vi "SequenceStatus.vi"(8 "error in (no error)":errorcluster, 9 "Motion Stopped":bool, 11 "VXMMotionManager in":refnum<class "VXMMotionManager.lvclass">) -> (0 "error out":errorcluster, 1 "last axis = True":bool, 3 "VXMMotionManager out":refnum<class "VXMMotionManager.lvclass">)   [LabVIEW 2019, in "VXMMotionManager.lvclass"]
doc: "change state from monitor motion to start next move\nincrement axis"
uses:
  VXMMotionManager.lvclass
  MoveAllAbsoluteStates.ctl
  VXMMotionManager.lvclass/VXMMotionManager.ctl
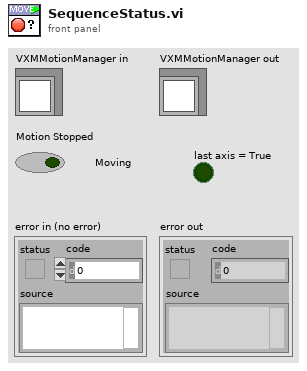
[diagram p1: front panel]
types:
  T1 = typedef "VXMMotionManager.lvclass/MoveAllAbsoluteStates.ctl" = enum16{"start next move", "wait motion end"}
  T2 = typedef "singleAxisMoveDef.ctl" = cluster{"mmWave Axis":T3, "eng. value":dbl}
  T3 = typedef "mmWaveAxis.ctl" = string
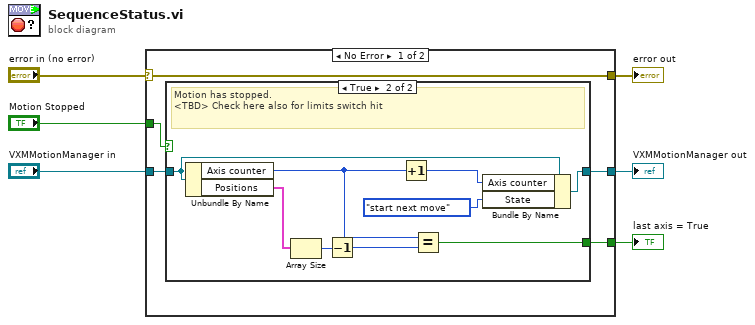
[diagram p0: block diagram]
diagram:
  n1 = case shown="No Error" "error in (no error)" {
    selector: "error in (no error)" -> [w11 w23]
    tunnel: [w11 w23] -> w3
    tunnel: [w10 w22] -> w4
    tunnel: "VXMMotionManager in" -> [w9 w22]
    tunnel: "Motion Stopped" -> [w8 _]
    tunnel: [w7 _] -> w1
    frame No Error {
      n2 = case shown="True" w8 {
        tunnel: [w12 w21] -> w10
        tunnel: w9 -> [w12 w20]
        tunnel: [_ w16] -> w7
        frame False {
          # "Still moving"
        }
        frame True {
          # "Motion has stopped.\n<TBD> Check here also for limits switch hit"
          n3 = Unbundle By Name(w20) -> ("Axis counter"=w17:i32, "Positions"=w15:T2[])
          n4 = Array Size(array=w15) -> (size(s)=w14:i32)
          n5 = Decrement(x=w14) -> (x-1=w13:i32)
          n6 = Increment(x=w17) -> (x+1=w19:i32)
          n7 = Equal?(x=w17, y=w13) -> (x = y?=w16:bool)
          n8 = Bundle By Name(cluster=w20, "Axis counter"=w19, "State"=MoveAllAbsoluteStates."start next move") -> (w21:refnum<class "VXMMotionManager.lvclass">)
        }
      }
    }
    frame Error {
    }
  }
  "error out" <- w3
  "VXMMotionManager out" <- w4
  "last axis = True" <- w1
